vi "Spawner.vi"() -> ()   [LabVIEW 2018]
panel:
  in  "stop":bool
  out "error out 2":errorcluster
  in  "error in (no error)":errorcluster
  in  "Spawn New":bool
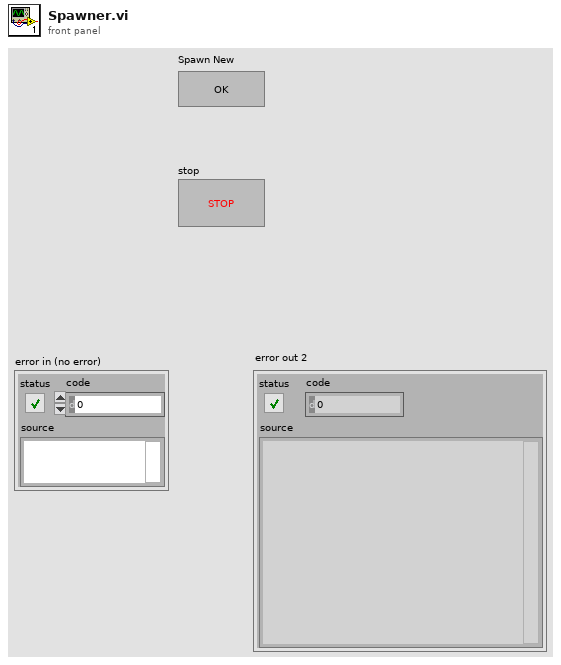
[diagram p1: front panel]
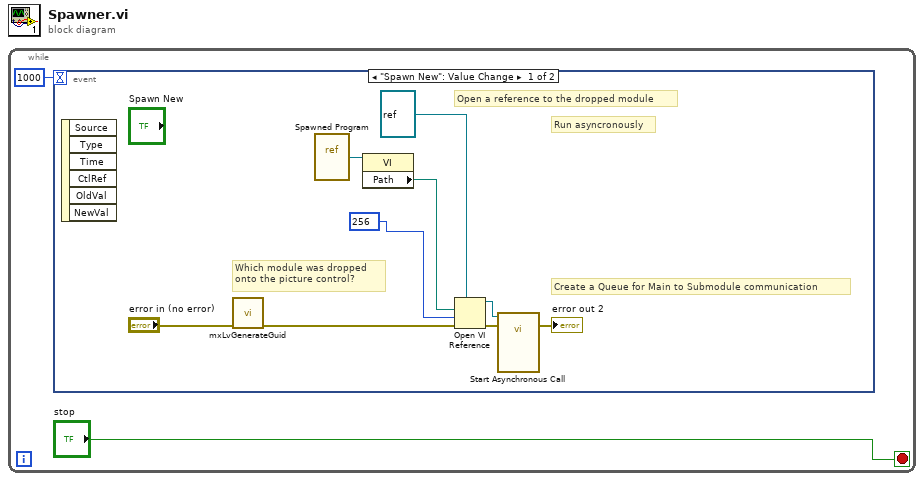
[diagram p0: block diagram]
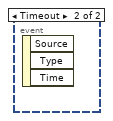
[diagram p2: hidden frame]
diagram:
  n1 = while {
    stop <- "stop" stop-if-true
    n2 = event shown="[0] \"Spawn New\": Value Change" {
      selector: _ -> [_ _]
      dyn-events: _ -> [_ _]
      timeout: 1000 -> [_ _]
      event "Spawn New": Value Change {
        # "Create a Queue for Main to Submodule communication"
        # "Run asyncronously"
        # "Open a reference to the dropped module"
        # "Which module was dropped\nonto the picture control?"
        n3 = event-data() -> ()  [unwired: 1 in, 6 out]
        n4 = call <resource>:"mxLvGenerateGuid.vi"("Error In"="error in (no error)") -> ("Error Out"=w6:errorcluster)  [unwired: 9 in, 1 out]
        n5 = vi-ref "Spawned Program.vi"() -> (w5:refnum<vi>)
        n6 = property class="VI"(reference=w5) -> ("Path"=w4:path)  [unwired: 1 in, 2 out]
        n7 = Open VI Reference(type specifier VI Refnum (for type only)=refnum<vi> refnum, vi path=w4, options=256, error in (no error)=w6) -> (vi reference=w8:refnum<vi>, error out=w9:errorcluster)  [unwired: 2 in]
        n8 = call-by-ref "Start Asynchronous Call"(reference=w8, error in=w9) -> (error out=→"error out 2":errorcluster)  [unwired: 12 in, 1 out]
      }
      event Timeout {
        n9 = event-data() -> ()  [unwired: 1 in, 3 out]
      }
    }
  }
